vi "fgv_serial_con_param.vi"(7 "serial_conn_set":bool, 8 "Error in":errorcluster, 9 "mode":string(combo)="Get", 10 "sweep_param_set":dbl[](array[numeric]), 11 "serial_port_set":refnum<visa-resource-name>="COM11") -> (0 "error out":errorcluster, 1 "sweep_param_get":dbl[](array[numeric]), 2 "scan_command_get":string, 3 "serial_port_get":refnum<visa-resource-name>="COM11", 5 "serial_conn_get":bool)   [LabVIEW 2025]
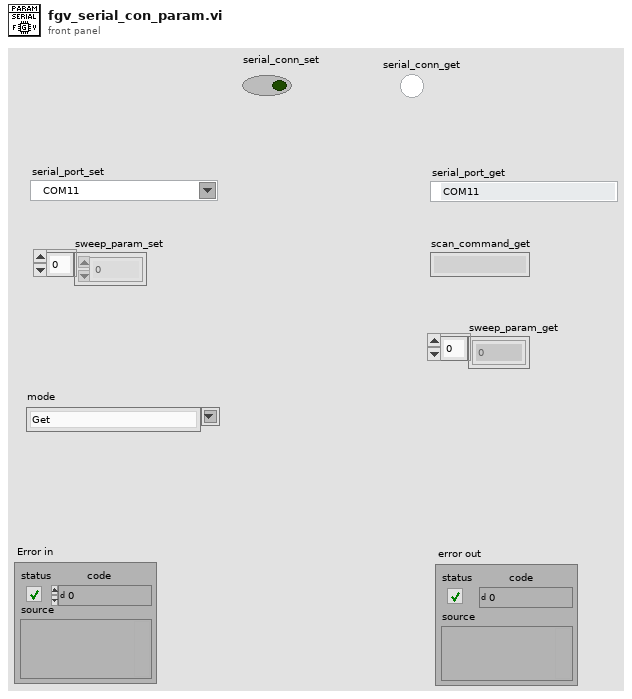
[diagram p1: front panel]
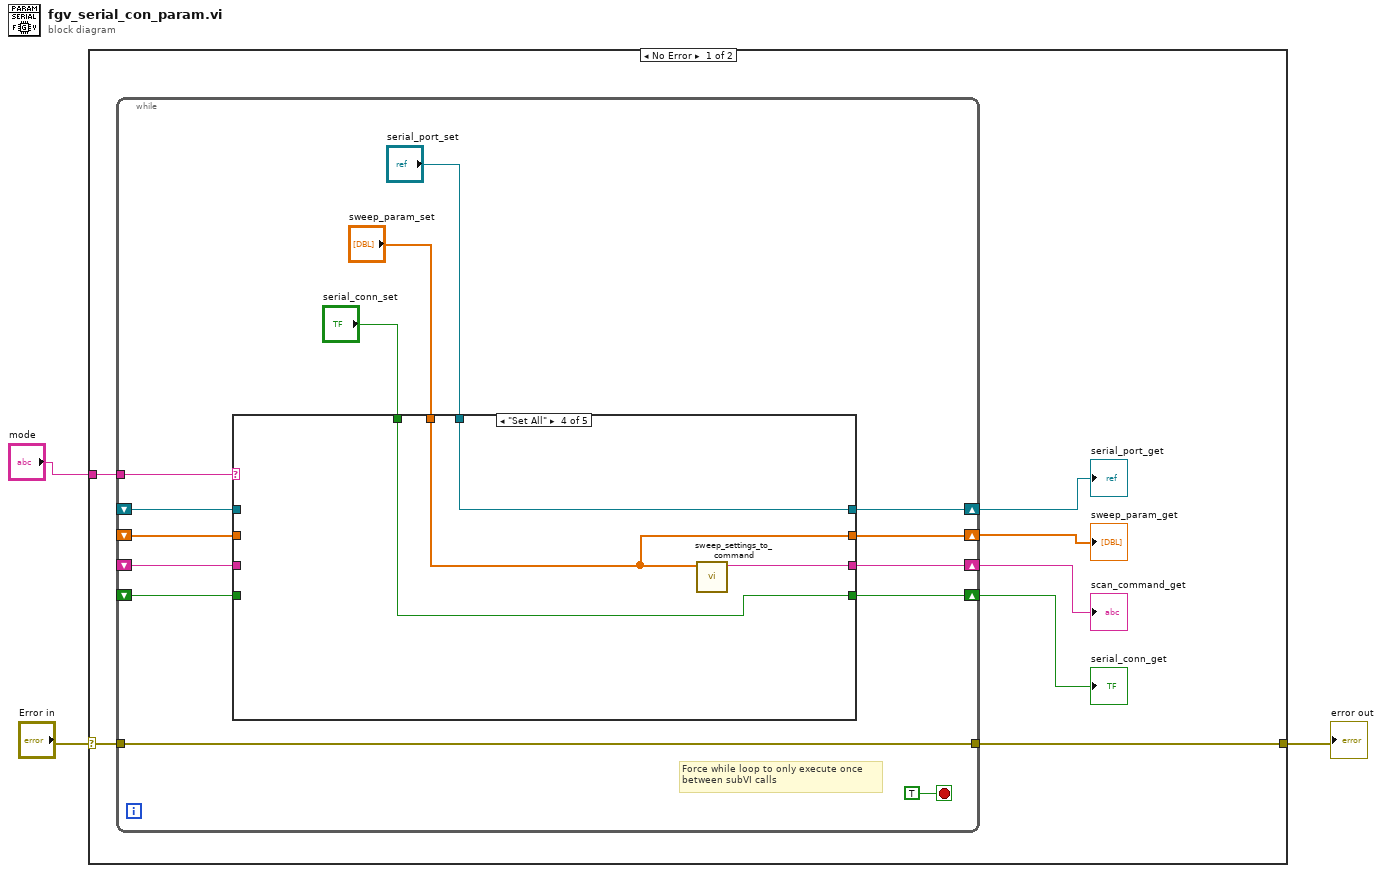
[diagram p0: block diagram]
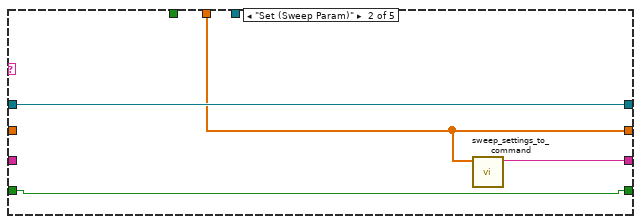
[diagram p3: hidden frame]
diagram:
  n1 = case shown="No Error" "Error in" {
    selector: "Error in" -> [w10 w45]
    tunnel: [w9 w45] -> w2
    tunnel: "mode" -> [w8 _]
    frame No Error {
      n2 = while {
        shift-right: [w22] -> w7
        shift-left: _ -> [w23]
        shift-right: [w21] -> w6
        shift-left: _ -> [w20]
        tunnel: w10 -> [w19]
        tunnel: [w19] -> w9
        tunnel: w8 -> [w18]
        shift-right: [w17] -> w5
        shift-left: _ -> [w16]
        shift-right: [w13] -> w4
        shift-left: _ -> [w11]
        stop <- TRUE stop-if-true
        # "Force while loop to only execute once\nbetween subVI calls"
        n3 = case shown="\"Set All\"" w18 {
          tunnel: w23 -> [_ w31 w36 _ w44]
          tunnel: [w26 w31 w36 w39 w44] -> w22
          tunnel: [w28 w30 w33 w38 w43] -> w21
          tunnel: w20 -> [w28 _ w33 _ w43]
          tunnel: [w27 w32 w34 w40 w42] -> w17
          tunnel: w16 -> [w27 _ w34 _ w42]
          tunnel: "serial_port_set" -> [w26 _ _ w39 _]
          tunnel: "sweep_param_set" -> [_ w30 _ w38 _]
          tunnel: [w25 w29 w35 w37 w41] -> w13
          tunnel: "serial_conn_set" -> [_ _ w35 w37 _]
          tunnel: w11 -> [w25 w29 _ _ w41]
          frame "Set (Serial Port)" {
          }
          frame "Set (Sweep Param)" {
            n4 = call "sweep_settings_to_command.vi"("sweep_param"=w30) -> ("scan_command"=w32:string)  [unwired: 10 in]
          }
          frame "Set (Serial Conn)" {
          }
          frame "Set All" {
            n5 = call "sweep_settings_to_command.vi"("sweep_param"=w38) -> ("scan_command"=w40:string)  [unwired: 10 in]
          }
          frame "Get", Default {
          }
        }
      }
      "serial_port_get" <- w7
      "sweep_param_get" <- w6
      "scan_command_get" <- w5
      "serial_conn_get" <- w4
    }
    frame Error {
      # "Case structure checks for errors - if there's an errorr, do nothing except pass the error back out"
    }
  }
  "error out" <- w2
